vi "practica 3 itiw31 tejada.vi"() -> ()   [LabVIEW 2018]
uses:
  <vilib>/express/express analysis/Spectral/Block/exnSpectralBlock spectral measurements RMS poly.vi
  <vilib>/express/express analysis/Spectral/Block/exnSpectralBlock spectral measurements RMS DDT.vi
  <vilib>/express/express analysis/Spectral/XNode/ExpressSpectralMeasurementsBlockNode.xnode
panel:
  out "Grafica en el dominio \nde la frecuencia":dynamicdata(graph)
  out "Grafica en el dominio \ndel tiempo":dynamicdata(graph)
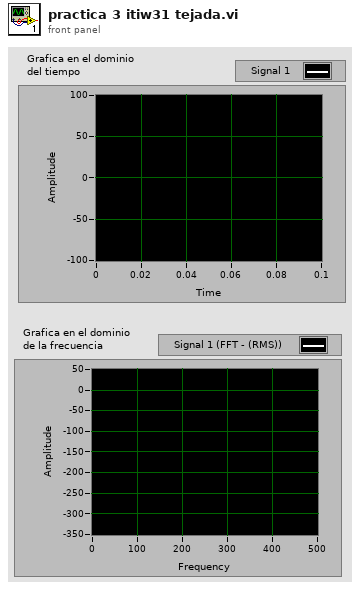
[diagram p1: front panel]
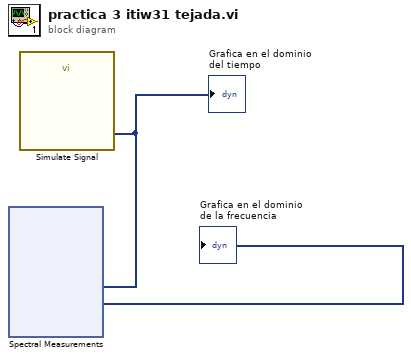
[diagram p0: block diagram]
diagram:
  n1 = call "Simulate Signal"() -> ("Signal 1"=w1:dynamicdata)  [unwired: 14 in, 1 out]
  "Grafica en el dominio \ndel tiempo" <- w1
  n2 = xnode "Spectral Measurements"("Signals"=w1) -> ("FFT - (RMS)"=→"Grafica en el dominio \nde la frecuencia":dynamicdata)  [unwired: 1 in, 2 out]
